vi "Control Panel.vi"() -> ()   [LabVIEW 2017]
uses:
  state-manager/State.ctl
  state-manager/Event.ctl
  <vilib>/Platform/TimedLoop/XDataNode/timing_clust.ctl
  <vilib>/Platform/TimedLoop/XDataNode/nitl_modes.ctl
  <vilib>/Platform/TimedLoop/XDataNode/wakeup.ctl
  Globals/Pose.vi
  Globals/Zig Zag Global.vi
  Globals/Gyro.vi
  Globals/Target Pose.vi
  Globals/Motor Speed Multiplier.vi
  <vilib>/Platform/TimedLoop/XDataNode/XDataNode.xnode
  <vilib>/Platform/TimedLoop/XDataNode/XDNodeRunTimeDep.lvlib
  <vilib>/myRIO/Express VI/Onboard IO/DI/DI Express VI.xnode
  <vilib>/myRIO/Instrument Drivers/Onboard IO/DIO/vis/Read.vi
  <vilib>/myRIO/Instrument Drivers/Onboard IO/DIO/DIO.lvlib
  <vilib>/myRIO/Common/Instrument Driver Framework/myRIO v1.0/DIO/typedefs/DIO Channels Enum.ctl
  <vilib>/myRIO/Common/Instrument Driver Framework/myRIO v1.0/DIO/typedefs/DIO Channels List.ctl
  <vilib>/myRIO/Common/Instrument Driver Framework/Utilities/typedefs/Generic FPGA Reference.ctl
  <vilib>/myRIO/Common/Instrument Driver Framework/Utilities/typedefs/myRIO v1.0 Reference.ctl
  <vilib>/myRIO/Common/Instrument Driver Framework/Utilities/typedefs/Hardware Version Enum.ctl
  <vilib>/myRIO/Common/Instrument Driver Framework/Utilities/typedefs/myRIO Generic Hardware Reference.ctl
  <vilib>/myRIO/Instrument Drivers/Onboard IO/DIO/typedefs/DIO Reference.ctl
  <vilib>/myRIO/Instrument Drivers/Onboard IO/DIO/vis/myRIO DIO Open.xnode
  <vilib>/myRIO/Common/Instrument Driver Framework/Utilities/vis/Is FPGA Ref Available.vi
  <vilib>/myRIO/Common/Instrument Driver Framework/myRIO v1.0/DIO/vis/myRIO v1.1 Open DIO.vi
  <vilib>/userdefined/High Color/nirio_resource_hc.ctl
panel:
  out "Red Button Pressed":bool
  out "Nothing shat itself in test":bool
  out "Event list":T1[](array[typedef])=[enum."Black Tape Crossed", enum."Ramp Passed", enum."Black Tape Crossed"]
  out "State list":T2[](array[typedef])
  out "Event Queue":T1[](array[typedef])=[enum."Black Tape Crossed"]
  in  "Pass In Event":bool
  in  "Manual Pass In Event":T1=enum."Start Button Pressed"
  in  "Speed":T3={"\nMoving speed"=0.4067796610169492, "Turning speed limit"=1.0296610169491527} {"Turning speed limit" scale=0.0..4.5; "Moving speed" scale=0.0..1.0}
  out "Current State":T2
  in  "Target Wall Distance":dbl=250.0
  in  "Stop Motors":bool
  out "LIDAR Data":cluster{dbl[], dbl[]}(graph)
  in  "LIDAR display update period (ms)":i64=500
  in  "Wall Left Indicator":bool=TRUE
  out "GYRO IS FUCKED":bool
  out "OH SHIT NO LIDAR DATA!!!":bool
  in  "OH SHIT, STOP":bool
  out "Gyro Bias":cluster{"X":dbl, "Y":dbl, "Z":dbl}={"X"=0.08609729920113632, "Y"=0.06396042865672143, "Z"=-0.2623400259994041}
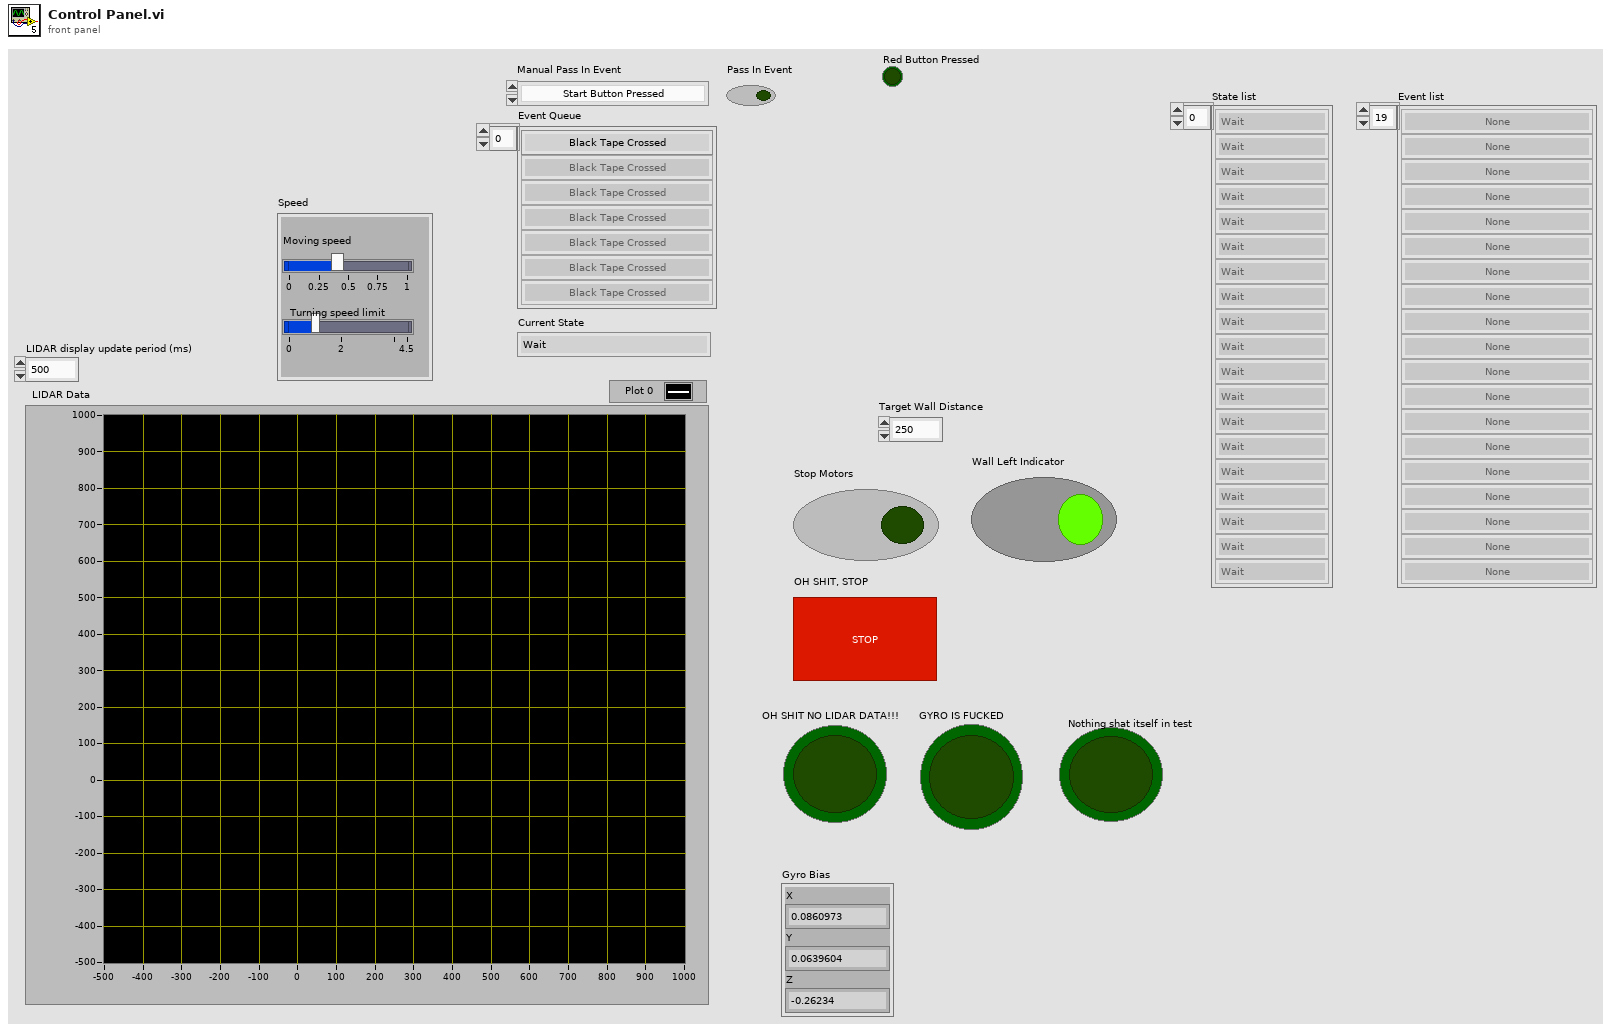
[diagram p1: front panel]
types:
  T1 = typedef "Event.ctl" = enum16{"None", "Zig Zag Finished", "Start Obstacle Avoidance", "Start Button Pressed", "Black & Yellow Tape Touched", "Black & Yellow Tape Passed", "Green Tape Crossed", "Red Tape Touched", "Rough Terrain Touched", "Black Tape Crossed", "Tape Edge Too Close", "Wall Too Close", "Rough Terrain Passed", "Ramp Passed", "Stop Button Pressed", "Recentered", "End Zone Wait Timed Out"}
  T2 = typedef "State.ctl" = enum16{"Wait", "Recenter", "Follow Wall", "Zig Zag", "Ramp", "Cross Rough Terrain", "Stagger Stop", "Obstacle Avoidance"}
  T3 = cluster{"\nMoving speed":dbl, "Turning speed limit":dbl}
  T4 = typedef "XDNodeRunTimeDep.lvlib/timing_clust.ctl" = cluster{"Expected End [f-1]":u64, "Actual End [f-1]":u64, "Finished Late? [f-1]":bool, "Expected End [i-1]":u64, "Actual End [i-1]":u64, "Finished Late? [i-1]":bool, "Expected Start [i]":u64, "Actual Start [i]":u64, "Expected Start [f]":u64, "Actual Start [f]":u64, "Source Name":string, "Structure Name":string, "Period":i64, "Deadline":i64, "Offset":i64, "Start":i64, "Priority":i32, "Timeout":i32, "Mode":T5, "Wakeup Reason":T6, "Error":errorcluster, "Source Type":string, "Secondary Source Type":string, "Global End Time":u64, "Global Start Time":u64, "Frame Duration":u64, "Iteration Duration":u64, "Assigned CPU":i32, "I/O Scan Engine Mode":u32}
  T5 = typedef "XDNodeRunTimeDep.lvlib/nitl_modes.ctl" = enum32{"No Change", "Process missed periods, maintain original phase", "Discard missed periods, maintain original phase", "Process missed periods, ignore original phase", "Discard missed periods, ignore original phase"}
  T6 = typedef "XDNodeRunTimeDep.lvlib/wakeup.ctl" = enum32{"Normal", "Aborted", "Asynchronous wakeup", "Timing source error", "Timed loop error", "Timeout"}
  T7 = typedef "DIO.lvlib/DIO Reference.ctl" = cluster{"myRIO Reference":T8, "DIO Channels List":T12}
  T8 = typedef "myRIO Generic Hardware Reference.ctl" = cluster{"myRIO Model":T9, "myRIO Hardware Reference":T10}
  T9 = typedef "Hardware Version Enum.ctl" = enum16{"Unknown", "myRIO-1900", "myRIO-1950", "roboRIO", "NI ELVIS RIO CM"}
  T10 = typedef "myRIO v1.0 Reference.ctl" = cluster{"Generic FPGA Reference":T11, "Allow multiple opens":bool}
  T11 = typedef "Generic FPGA Reference.ctl" = refnum<k20>
  T12 = typedef "DIO Channels List.ctl" = T13[]
  T13 = typedef "DIO Channels Enum.ctl" = enum16{"Not Connected", "C/DIO0", "C/DIO1", "C/DIO2", "C/DIO3", "C/DIO4", "C/DIO5", "C/DIO6", "C/DIO7", "A/DIO0", "A/DIO1", "A/DIO2", "A/DIO3", "A/DIO4", "A/DIO5", "A/DIO6", "A/DIO7", "A/DIO8", "A/DIO9", "A/DIO10", "A/DIO11", "A/DIO12", "A/DIO13", "A/DIO14", "A/DIO15", "B/DIO0", "B/DIO1", "B/DIO2", "B/DIO3", "B/DIO4", "B/DIO5", "B/DIO6", "B/DIO7", "B/DIO8", "B/DIO9", "B/DIO10", "B/DIO11", "B/DIO12", "B/DIO13", "B/DIO14", "B/DIO15", "LED0", "LED1", "LED2", "LED3", "Button0", "DIO/DIO0", "DIO/DIO1", "DIO/DIO2", "DIO/DIO3", "DIO/DIO4", "DIO/DIO5", "DIO/DIO6", "DIO/DIO7", "DIO/DIO8", "DIO/DIO9", "SPI/CS0", "SPI/CS1", "SPI/CS2", "SPI/CS3", "LED RADIO (Green)", "LED RADIO (Red)", "LED COMM (Green)", "LED COMM (Red)", "LED MODE (Green)", "LED MODE (Red)"}
  T14 = typedef "nirio_resource_hc.ctl" = tag
  T15 = typedef "IMAQdx.ctl" = refnum<k21>
  T16 = typedef "I2C.lvlib/I2C Reference.ctl" = cluster{"myRIO Reference":T8, "I2C Channels Enum":T17, "I2C Configuration":T18}
  T17 = typedef "I2C Channels Enum.ctl" = enum16{"Not Connected", "A/I2C", "B/I2C", "I2C/I2C"}
  T18 = typedef "I2C.lvlib/I2C Configuration.ctl" = cluster{"I2C Transfer Rate":T19}
  T19 = typedef "I2C.lvlib/I2C Transfer Rate.ctl" = enum16{"Standard mode (100 kbps)", "Fast mode (400 kbps)"}
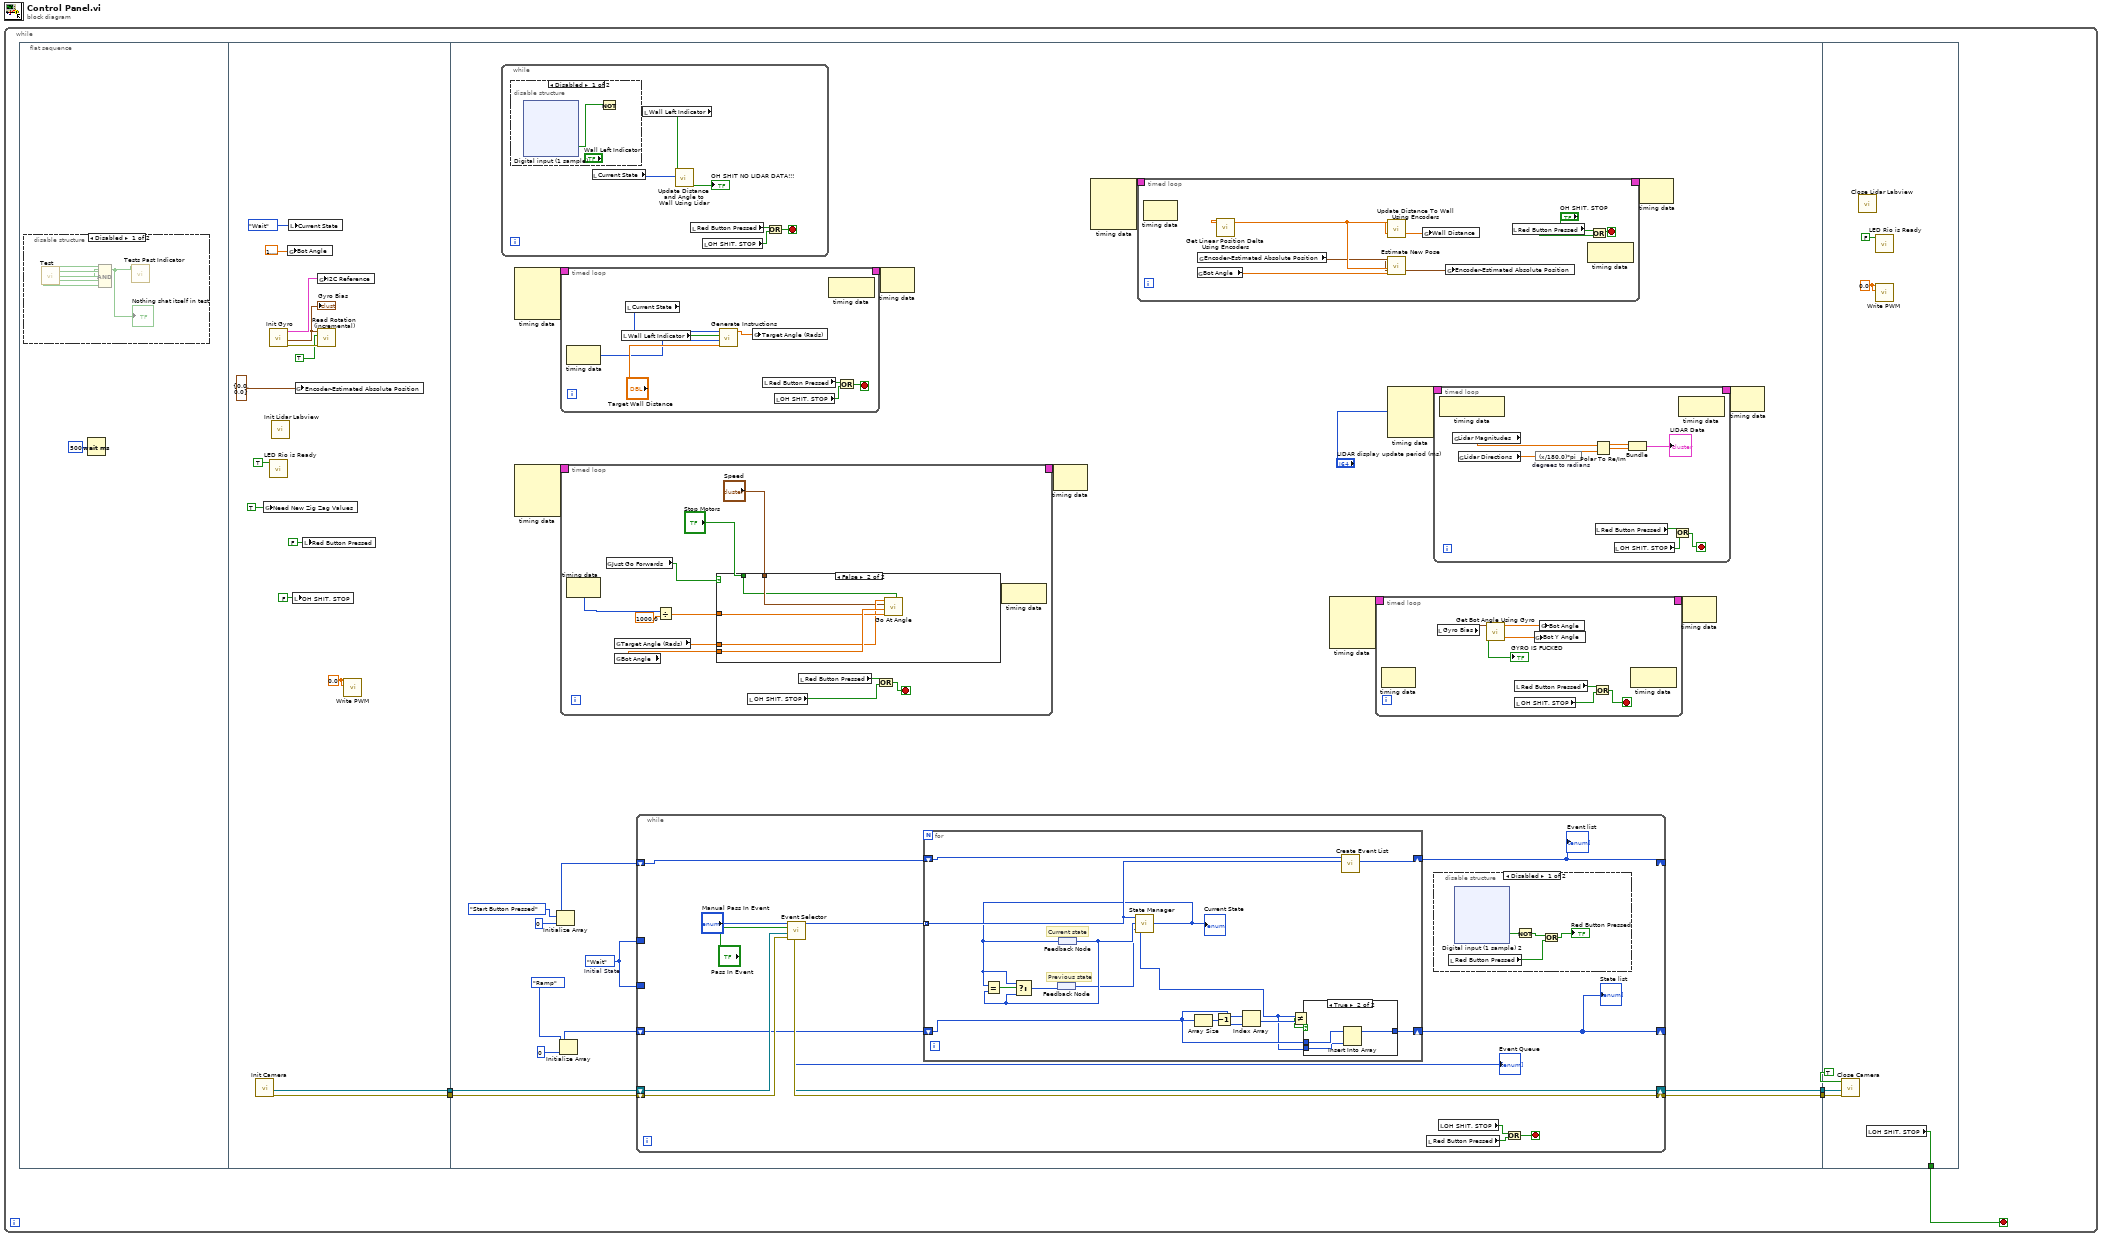
[diagram p0: block diagram]
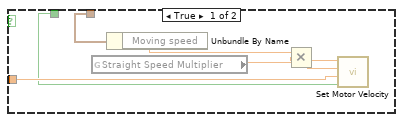
[diagram p5: hidden frame]
diagram:
  n1 = while {
    stop <- w1 stop-if-true
    n2 = flat-sequence {
      tunnel: [w23] -> w4
      tunnel: [w22] -> w5
      tunnel: w5 -> [w41]
      tunnel: [w40] -> w3
      tunnel: [w38] -> w2
      tunnel: w4 -> [w39]
      tunnel: w3 -> [w246]
      tunnel: w2 -> [w245]
      tunnel: [w242] -> w1
      frame #0 {
        n3 = disable-structure shown="Disabled" {
          frame Disabled {
            n4 = call "Test.vi"() -> ("Encoders Working\n(backwards)"=w12:bool, "Encoders Working\n(forwards)"=w11:bool, "Event Passed In Correctly"=w10:bool, "LIDAR Gets Data"=w9:bool, "Gyro Angle Correct 2"=w8:bool)  [unwired: 11 in]
            n5 = Compound Arithmetic op=AND(w12, w11, w10, w9, w8) -> (w7:bool)
            "Nothing shat itself in test" <- w7
            n6 = call "Tests Past Indicator.vi"("Test Past"=w7) -> ()  [unwired: 11 in]
          }
          frame Enabled {
          }
        }
        n7 = Wait (ms)(milliseconds to wait=u32 500) -> ()  [unwired: 1 out]
      }
      frame #1 {
        w18 = 0.0 ("Left")
        n8 = call "Init Camera.vi"() -> ("error out"=w23:errorcluster, "session out"=w22:T15)  [unwired: 9 in]
        n9 = global write "Zig Zag Global.vi" "Need New Zig Zag Values"(TRUE ("Zig Zag Finished")) -> ()
        n10 = call "Init Gyro.vi"() -> ("error out"=w16:errorcluster, "Gyro Bias"=w14:cluster{"X":dbl, "Y":dbl, "Z":dbl}, "I2C Ref Out"=w17:T16)  [unwired: 9 in]
        "Gyro Bias" <- w14
        n11 = call "LED Rio is Ready.vi"("Rio is ready"=TRUE) -> ()  [unwired: 11 in]
        n12 = call "Init Lidar Labview.vi"() -> ()  [unwired: 11 in, 1 out]
        n13 = global write "Pose.vi" "Bot Angle"(1.5707963267948966) -> ()
        n14 = local write "Current State"(State."Wait" ("Current State")) -> ()
        n15 = local write "OH SHIT, STOP"(FALSE ("OH SHIT, STOP")) -> ()
        n16 = global write "Pose.vi" "Encoder-Estimated Absolute Position"(cluster{"X":dbl, "Y":dbl} {"X"=0.0, "Y"=0.0} ("Encoder-Estimated Absolute Position")) -> ()
        n17 = local write "Red Button Pressed"(FALSE ("Red Button Pressed")) -> ()
        n18 = global write "Gyro.vi" "I2C Reference"(w17) -> ()
        n19 = call "Read Rotation (incremental).vi"("error in (no error)"=w16, "reset"=TRUE, "Gyro bias"=w14) -> ()  [unwired: 7 in, 2 out]
        n20 = call "Write PWM.vi"("Left"=w18, "Right"=w18) -> ()  [unwired: 8 in]
      }
      frame #2 {
        w29 = State."Wait"  # Initial State
        n21 = while {
          stop <- w187 stop-if-true
          n22 = disable-structure shown="Disabled" {
            frame Disabled {
              n23 = xnode "Digital input (1 sample)"() -> ("Switch for Left Right (A/DIO2 (Pin 15))"=w193:bool)  [unwired: 1 in, 1 out]
              n24 = Not(x=w193) -> (.not. x?=w192:bool)
            }
            frame Enabled {
            }
          }
          n25 = local read "Current State"() -> (w190:T2)
          n26 = local read "Wall Left Indicator"() -> (w186:bool)
          n27 = call "Update Distance and Angle to Wall Using Lidar.vi"("Current State"=w190, "Wall Left?"=w186) -> ("OH SHIT NO LIDAR DATA!!!"=→"OH SHIT NO LIDAR DATA!!!":bool)  [unwired: 9 in]
          n28 = local read "Red Button Pressed"() -> (w189:bool)
          n29 = local read "OH SHIT, STOP"() -> (w188:bool)
          n30 = Or(x=w189, y=w188) -> (x .or. y?=w187:bool)
        }
        n31 = node-c288() -> (w43:T4)  [unwired: 4 in]
        n32 = node-c288() -> (w37:T4)  [unwired: 4 in]
        n33 = Initialize Array(Event."Start Button Pressed" ("Event"), 0 ("dimension size")) -> (w30:T1[])
        n34 = Initialize Array(State."Ramp" ("y"), 0 ("dimension size")) -> (w33:T2[])
        n35 = timed-loop {
          timing: w43 -> [_]
          timing-out: [_] -> w42
          stop <- w159 stop-if-true
          n36 = node-c288() -> (w163:i64)  [unwired: 1 in]
          n37 = local read "Wall Left Indicator"() -> (w164:bool)
          n38 = local read "Current State"() -> (w162:T2)
          n39 = call "Generate Instructions.vi"("State"=w162, "Wall Left?"=w164, "dt"=w163, "Target Distance"="Target Wall Distance") -> ("Target Angle"=w161:dbl)  [unwired: 6 in]
          n40 = global write "Target Pose.vi" "Target Angle (Rads)"(w161) -> ()
          n41 = local read "Red Button Pressed"() -> (w160:bool)
          n42 = local read "OH SHIT, STOP"() -> (w158:bool)
          n43 = node-c288() -> ()  [unwired: 1 in, 1 out]
          n44 = Or(x=w160, y=w158) -> (x .or. y?=w159:bool)
        }
        n45 = timed-loop {
          timing: w37 -> [_]
          timing-out: [_] -> w36
          stop <- w131 stop-if-true
          n46 = node-c288() -> (w140:i64)  [unwired: 1 in]
          n47 = global read "Pose.vi" "Just Go Forwards"() -> (w134:bool)
          n48 = global read "Target Pose.vi" "Target Angle (Rads)"() -> (w135:dbl)
          n49 = global read "Pose.vi" "Bot Angle"() -> (w139:dbl)
          n50 = Divide(x=w140, y=1000.0) -> (x/y=w138:dbl)
          n51 = case shown="False" w134 {
            tunnel: w139 -> [_ w152]
            tunnel: w138 -> [w147 w151]
            tunnel: "Stop Motors" -> [w146 w148]
            tunnel: "Speed" -> [w145 w149]
            tunnel: w135 -> [_ w150]
            frame True {
              n52 = global read "Motor Speed Multiplier.vi" "Straight Speed Multiplier"() -> (w142:dbl)
              n53 = Unbundle By Name(w145) -> ("Moving speed"=w144:dbl)
              n54 = Multiply(x=w144, y=w142) -> (x*y=w143:dbl)
              n55 = call "Set Motor Velocity.vi"("Disable motors"=w146, "dt"=w147, "Right motor speed rev/s"=w143, "Left motor speed rev/s"=w143) -> ()  [unwired: 8 in]
            }
            frame False {
              n56 = call "Go At Angle.vi"("Target Angle"=w150, "Speed"=w149, "Bot Angle"=w152, "dt"=w151, "Stop motors"=w148) -> ()  [unwired: 6 in]
            }
          }
          n57 = local read "OH SHIT, STOP"() -> (w132:bool)
          n58 = local read "Red Button Pressed"() -> (w133:bool)
          n59 = Or(x=w133, y=w132) -> (x .or. y?=w131:bool)
          n60 = node-c288() -> ()  [unwired: 1 in, 1 out]
        }
        n61 = while {
          shift-right: [w71] -> w38
          shift-left: w39 -> [w73]
          shift-right: [w70] -> w40
          shift-left: w41 -> [w72]
          shift-right: [w65] -> _
          shift-left: w33 -> [w66]
          shift-right: [w64] -> _
          shift-left: w30 -> [w63]
          border: w29 -> [_]
          border: w29 -> [_]
          stop <- w60 stop-if-true
          n62 = call "Event Selector.vi"("Error In"=w73, "Session In"=w72, "Pass In Event"="Pass In Event", "Manual Pass In Event"="Manual Pass In Event") -> ("Error Out"=w71:errorcluster, "Session Out"=w70:T15, "Event Queue"=w67:T1[])  [unwired: 5 in]
          "Event Queue" <- w67
          n63 = for {
            tunnel: w67 -> [w119] mode=indexing
            shift-right: [w121] -> w65
            shift-left: w66 -> [w122]
            shift-right: [w118] -> w64
            shift-left: w63 -> [w120]
            # "Previous state"
            # "Current state"
            n64 = feedback #1() -> (w114:T2)
            n65 = feedback #2() -> (w115:T2)
            n66 = call "State Manager.vi"("Previous State"=w114, "Current State"=w115, "Event"=w119) -> ("Next State"=w113:T2)
            "Current State" <- w113
            n67 = Equal?(x=w113, y=w115) -> (x = y?=w117:bool)
            n68 = Select(t=w113, s=w117, f=w115) -> (s? t:f=w116:T2)
            n69 = feedback-in #1(w116) -> ()
            n70 = feedback-in #2(w113) -> ()
            n71 = Array Size(array=w122) -> (size(s)=w126:i32)
            n72 = Decrement(x=w126) -> (x-1=w125:i32)
            n73 = Index Array(array=w122, index=w125) -> (element=w124:T2)
            n74 = Not Equal?(x=w113, y=w124) -> (x != y?=w123:bool)
            n75 = case shown="True" w123 {
              tunnel: w122 -> [w127 w130]
              tunnel: w113 -> [_ w129]
              tunnel: [w127 w128] -> w121
              frame False {
              }
              frame True {
                n76 = Insert Into Array(array=w130, new element=w129) -> (w128:T2[])  [unwired: 1 in]
              }
            }
            n77 = call "Create Event List.vi"("Event Outcome"=w119, "Array in"=w120) -> ("Array out"=w118:T1[])  [unwired: 9 in]
          }
          "State list" <- w65
          "Event list" <- w64
          n78 = local read "Red Button Pressed"() -> (w61:bool)
          n79 = disable-structure shown="Disabled" {
            frame Disabled {
              n80 = local read "Red Button Pressed"() -> (w74:bool)
              n81 = xnode "Digital input (1 sample) 2"() -> ("A/DIO0 (Pin 11)"=w77:bool)  [unwired: 1 in, 1 out]
              n82 = Not(x=w77) -> (.not. x?=w76:bool)
              n83 = Or(x=w76, y=w74) -> (x .or. y?=→"Red Button Pressed":bool)
            }
            frame Enabled {
            }
          }
          n84 = local read "OH SHIT, STOP"() -> (w62:bool)
          n85 = Or(x=w62, y=w61) -> (x .or. y?=w60:bool)
        }
        n86 = node-c288(w42) -> ()  [unwired: 1 out]
        n87 = node-c288(w36) -> ()  [unwired: 1 out]
        n88 = node-c288() -> (w48:T4)  [unwired: 4 in]
        n89 = timed-loop {
          timing: w48 -> [_]
          timing-out: [_] -> w47
          stop <- w229 stop-if-true
          n90 = node-c288() -> ()  [unwired: 1 in, 1 out]
          n91 = global read "Pose.vi" "Bot Angle"() -> (w234:dbl)
          n92 = global read "Pose.vi" "Encoder-Estimated Absolute Position"() -> (w233:cluster{"X":dbl, "Y":dbl})
          n93 = call "Get Linear Position Delta Using Encoders.vi"() -> ("Change in Linear Position (mm)"=w235:dbl)  [unwired: 11 in]
          n94 = call "Update Distance To Wall Using Encoders.vi"("Linear Distance Travelled (mm)"=w235) -> ("Wall Distance"=w236:dbl)  [unwired: 10 in]
          n95 = call "Estimate New Pose.vi"("Bot Angle (rad)"=w234, "Linear Distance Travelled (mm)"=w235, "Current Absolute Position"=w233) -> ("Updated Absolute Position"=w232:cluster{"X":dbl, "Y":dbl})  [unwired: 8 in]
          n96 = global write "Pose.vi" "Wall Distance"(w236) -> ()
          n97 = global write "Pose.vi" "Encoder-Estimated Absolute Position"(w232) -> ()
          n98 = local read "Red Button Pressed"() -> (w230:bool)
          n99 = node-c288() -> ()  [unwired: 1 in, 1 out]
          n100 = Or(x="OH SHIT, STOP", y=w230) -> (x .or. y?=w229:bool)
        }
        n101 = node-c288() -> (w28:T4)  [unwired: 4 in]
        n102 = timed-loop {
          timing: w28 -> [_]
          timing-out: [_] -> w27
          stop <- w49 stop-if-true
          n103 = node-c288() -> ()  [unwired: 1 in, 1 out]
          n104 = local read "Gyro Bias"() -> (w53:cluster{"X":dbl, "Y":dbl, "Z":dbl})
          n105 = call "Get Bot Angle Using Gyro.vi"("Gyro bias"=w53) -> ("Y Rotation (rads)"=w52:dbl, "GYRO IS FUCKED"=→"GYRO IS FUCKED":bool, "Z Rotation (rads)"=w55:dbl)  [unwired: 7 in, 1 out]
          n106 = local read "Red Button Pressed"() -> (w51:bool)
          n107 = local read "OH SHIT, STOP"() -> (w50:bool)
          n108 = global write "Pose.vi" "Bot Y Angle"(w52) -> ()
          n109 = global write "Pose.vi" "Bot Angle"(w55) -> ()
          n110 = Or(x=w51, y=w50) -> (x .or. y?=w49:bool)
          n111 = node-c288() -> ()  [unwired: 1 in, 1 out]
        }
        n112 = node-c288("LIDAR display update period (ms)") -> (w46:T4)  [unwired: 3 in]
        n113 = timed-loop {
          timing: w46 -> [_]
          timing-out: [_] -> w45
          stop <- w171 stop-if-true
          n114 = node-c288() -> ()  [unwired: 1 in, 1 out]
          n115 = global read "Pose.vi" "Lidar Magnitudes"() -> (w179:dbl[])
          n116 = global read "Pose.vi" "Lidar Directions"() -> (w174:dbl[])
          n117 = expression code="(x/180.0)*pi" "degrees to radians"(w174) -> (w175:dbl[])
          n118 = Polar To Re/Im(2:w175, 3:w179) -> (0:w177:dbl[], 1:w178:dbl[])
          n119 = local read "Red Button Pressed"() -> (w173:bool)
          n120 = local read "OH SHIT, STOP"() -> (w172:bool)
          n121 = Bundle(w178, w177) -> (→"LIDAR Data":cluster{dbl[], dbl[]})  [unwired: 1 in]
          n122 = Or(x=w173, y=w172) -> (x .or. y?=w171:bool)
          n123 = node-c288() -> ()  [unwired: 1 in, 1 out]
        }
        n124 = node-c288(w47) -> ()  [unwired: 1 out]
        n125 = node-c288(w27) -> ()  [unwired: 1 out]
        n126 = node-c288(w45) -> ()  [unwired: 1 out]
      }
      frame #3 {
        w241 = 0.0 ("Left")
        n127 = call "Close Camera.vi"("error in"=w245, "Session In"=w246, "stop"=TRUE) -> ()  [unwired: 7 in, 2 out]
        n128 = call "Close Lidar Labview.vi"() -> ()  [unwired: 11 in, 1 out]
        n129 = local read "OH SHIT, STOP"() -> (w242:bool)
        n130 = call "LED Rio is Ready.vi"("Rio is ready"=FALSE) -> ()  [unwired: 11 in]
        n131 = call "Write PWM.vi"("Left"=w241, "Right"=w241) -> ()  [unwired: 8 in]
      }
    }
  }
